vi "Tosca-Strip Mandatory DI.vi"(7 "Digital Signals":string[](array[string]), 11 "Lines":i32[](array[numeric])) -> (8 "Filtered DI":string[](array[string]), 14 "Required":string[](array[string]), 15 "Filtered Lines":i32[](array[numeric]))   [LabVIEW 2020]
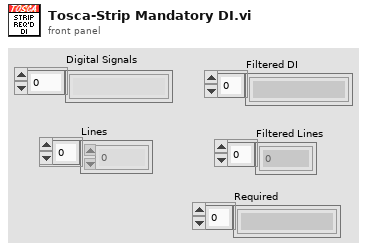
[diagram p1: front panel]
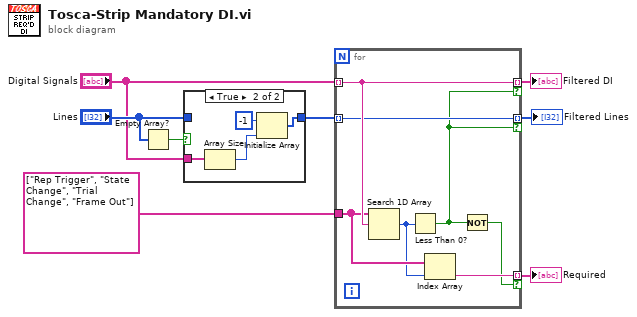
[diagram p0: block diagram]
diagram:
  n1 = Empty Array?(array="Lines") -> (empty?=w4:bool)
  n2 = case shown="True" w4 {
    tunnel: "Lines" -> [w9 _]
    tunnel: [w9 w12] -> w3
    tunnel: "Digital Signals" -> [_ w10]
    frame False {
    }
    frame True {
      n3 = Array Size(array=w10) -> (size(s)=w11:i32)
      n4 = Initialize Array(-1, w11) -> (w12:i32[])
    }
  }
  n5 = for {
    tunnel: "Digital Signals" -> [w20] mode=indexing
    tunnel: string[] ["Rep Trigger", "State Change", "Trial Change", "Frame Out"] -> [w17]
    tunnel: [w20] -> w7 mode=indexing if=w18
    tunnel: w3 -> [w19] mode=indexing
    tunnel: [w19] -> w6 mode=indexing if=w18
    tunnel: [w15] -> w1 mode=indexing if=w14
    n6 = Search 1D Array(1D array=w17, element=w20) -> (index of element=w16:i32)  [unwired: 1 in]
    n7 = Less Than 0?(x=w16) -> (x < 0?=w18:bool)
    n8 = Index Array(array=w17, index=w16) -> (element=w15:string)
    n9 = Not(x=w18) -> (.not. x?=w14:bool)
  }
  "Filtered DI" <- w7
  "Filtered Lines" <- w6
  "Required" <- w1
